vi "ni579x Construct Command Set Amplifier.vi"(0 "Register Bus":refnum<class "ni579x Register Bus v1 Host.lvclass">=refnum, 1 "scope":string, 5 "enabled?":bool=TRUE, 11 "Error In":errorcluster) -> (4 "Register Bus (out)":refnum<class "ni579x Register Bus v1 Host.lvclass">, 6 "User Command":T1 {"User Command ID" items=["Set Clock Select"=0, "Set CLK OUT Source"=1, "DAC Sync User Start"=2, "DAC Sync User End"=3, "Enable Baseband Amp"=5, "Set Rx Attenuation Pre-LNA"=7, "Set Rx Attenuation Post-LNA"=8, "Set Tx Attenuation"=9, "Set LO Filter"=32, "Set Front End Filter"=33, "Enable LO"=34, "Set Routing Mux"=37, "Read Current Rev Lower"=240, "Read Current Rev Upper"=241, "Read Oldest Compat Rev Lower"=242, "Read Oldest Compat Rev Upper"=243, "Re-Initialize"=255]; "User Data 1" format="%x"; "User Data 0" format="%x"}, 15 "Error Out":errorcluster)   [LabVIEW 2015]
uses:
  <instrlib>/ni579x/Register Bus/v1/Host/ni579x Register Bus v1 Host.lvclass
  <instrlib>/ni579x/Config/v1/Shared/Types/ni579x User Command.ctl
  <instrlib>/ni579x/Config/v1/Shared/Types/ni579x User Command ID.ctl
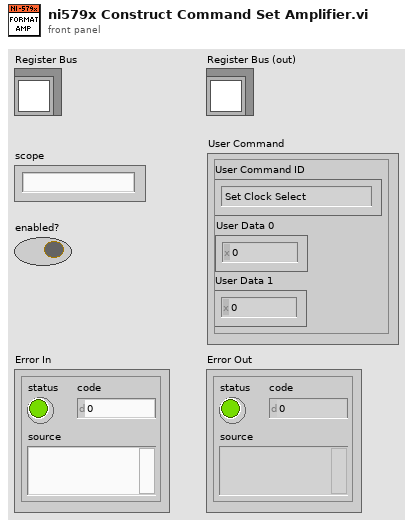
[diagram p1: front panel]
types:
  T1 = typedef "ni579x User Command.ctl" = cluster{"User Data 0":u8, "User Data 1":u8, "User Command ID":T2}
  T2 = typedef "ni579x User Command ID.ctl" = u8
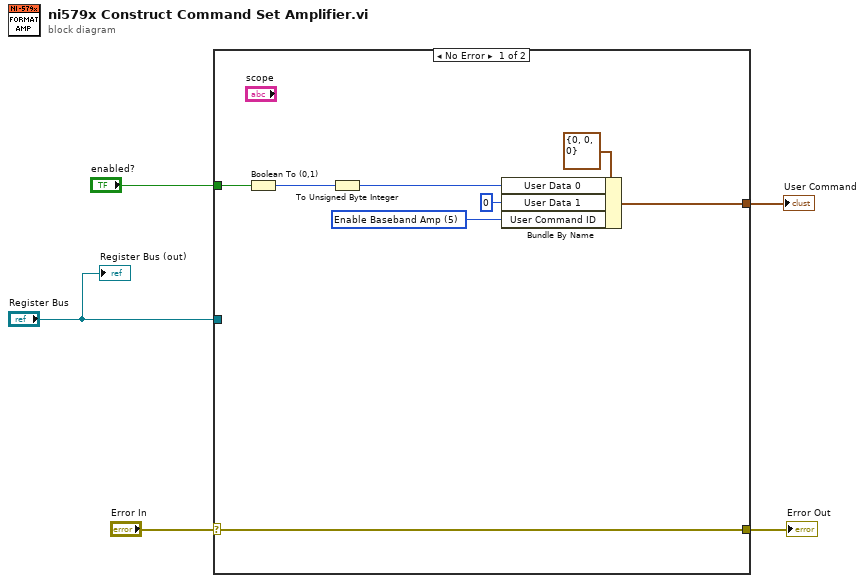
[diagram p0: block diagram]
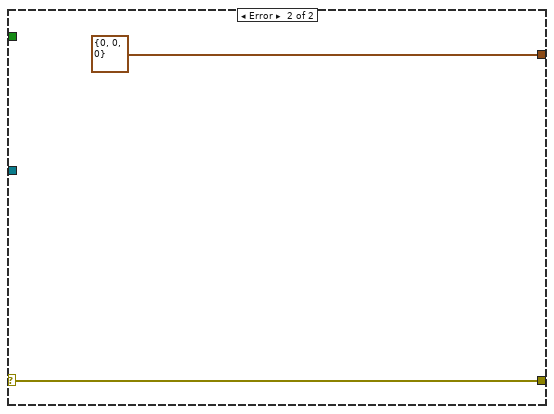
[diagram p2: hidden frame]
diagram:
  n1 = case shown="No Error" "Error In" {
    selector: "Error In" -> [w12 w15]
    tunnel: [w12 w15] -> w4
    tunnel: "Register Bus" -> [_ _]
    tunnel: "enabled?" -> [w9 _]
    tunnel: [w13 T1 {"User Data 0"=0, "User Data 1"=0, "User Command ID"=0} ("User Command")] -> w1
    frame No Error {
      w6 = T2 5 items=["Set Clock Select"=0, "Set CLK OUT Source"=1, "DAC Sync User Start"=2, "DAC Sync User End"=3, "Enable Baseband Amp"=5, "Set Rx Attenuation Pre-LNA"=7, "Set Rx Attenuation Post-LNA"=8, "Set Tx Attenuation"=9, "Set LO Filter"=32, "Set Front End Filter"=33, "Enable LO"=34, "Set Routing Mux"=37, "Read Current Rev Lower"=240, "Read Current Rev Upper"=241, "Read Oldest Compat Rev Lower"=242, "Read Oldest Compat Rev Upper"=243, "Re-Initialize"=255] ("User Command ID")
      n2 = Boolean To (0,1)(Boolean=w9) -> (0, 1=w8:i16)
      n3 = To Unsigned Byte Integer(number=w8) -> (unsigned 8bit integer=w7:u8)
      n4 = Bundle By Name(cluster=T1 {"User Data 0"=0, "User Data 1"=0, "User Command ID"=0} ("User Command"), "User Data 0"=w7, "User Data 1"=u8 0, "User Command ID"=w6) -> (w13:T1)
    }
    frame Error {
    }
  }
  "Error Out" <- w4
  "User Command" <- w1
  "Register Bus (out)" <- "Register Bus"
